vi "Actor Core.vi"(8 "error in":errorcluster, 11 "Sweeper  in":refnum<class "Sweeper.lvclass">) -> (0 "error out":errorcluster, 3 "Actor out":refnum<class "Actor.lvclass">)   [LabVIEW 2018, in "Sweeper.lvclass"]
doc: "(<B>Filename</B>: Actor Framework.lvlib:Actor.lvclass:Actor Core.vi)\n\nReceives messages to the actor, reacts to them, and initiates any error handling that may shut the actor down.\n\nDescendant classes may override this VI to append parallel tasks for the actor to complete while it handles messages. Overrides use the Call Parent Method node."
uses:
  Sweeper.lvclass
  C:/github/LabActor/Template Module/Template Module.lvclass
  C:/Program Files/National Instruments/LabVIEW 2018/vi.lib/ActorFramework/Actor/Actor.lvclass
  <vilib>/ActorFramework/Actor/Actor.lvclass
  NHMFL_Core/Libraries/Instruments/Controls/Set Output.ctl
  NHMFL_Core/Libraries/Instruments/Controls/Sweep Action.ctl
  Template Module/Template Module.lvclass/Template Module.ctl
  <vilib>/ActorFramework/Actor/Actor.lvclass/Actor.ctl
  <vilib>/ActorFramework/Message Enqueuer/Message Enqueuer.lvclass/Message Enqueuer.ctl
  NHMFL_Core/Libraries/Instruments/Results/Set Sweep/Set Sweep.lvclass
  C:/github/NHMFL_Core/Libraries/Utilities/Output Value/Output Value.lvclass
  Instrument Actor Messages/Set Output Msg/Set Output Msg.lvclass/Set Output Msg.ctl
  Template Module/Read stop event.vi
  <vilib>/ActorFramework/Message Enqueuer/Init from Existing Queue.vi
  <vilib>/ActorFramework/Message Enqueuer/Enqueue.vi
  Instrument Actor Messages/Set Output Msg/Set Output Msg.lvclass
  C:/Program Files/National Instruments/LabVIEW 2018/vi.lib/ActorFramework/Message/Message.lvclass
  <vilib>/ActorFramework/Message Priority Queue/Priority Enqueue.vi
  Instrument Actor/Instrument Actor.lvclass
  <vilib>/ActorFramework/Message Enqueuer/Message Enqueuer.lvclass
panel:
  in  "Go Button":bool
  out "Name":string
  in  "Configuration":T1={"Set point"=0.0, "Sweep rate"=0.0, "Sweep action"=enum."To set point"}
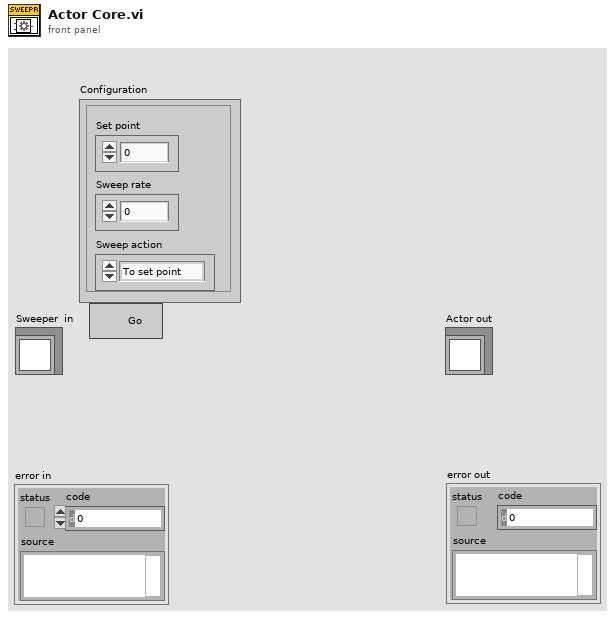
[diagram p1: front panel]
types:
  T1 = typedef "Set Output.ctl" = cluster{"Set point":dbl, "Sweep rate":dbl, "Sweep action":T2}
  T2 = typedef "Sweep Action.ctl" = enum16{"Hold", "To set point", "To zero", "Clamp"}
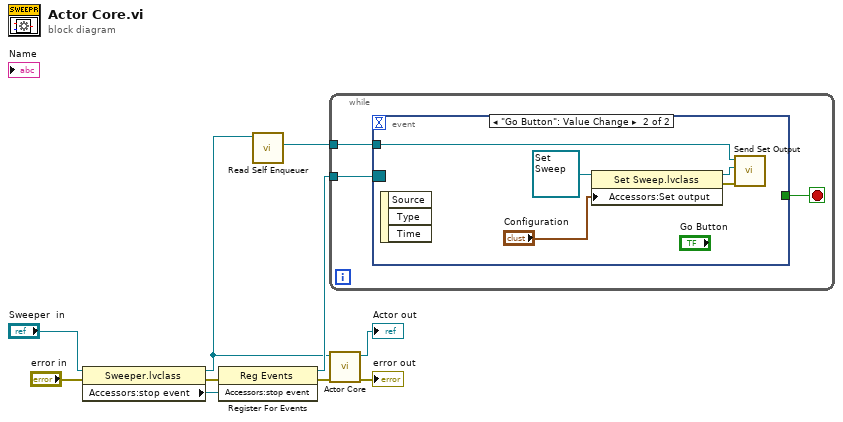
[diagram p0: block diagram]
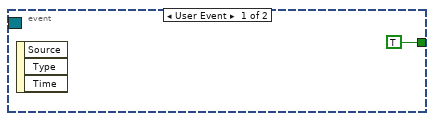
[diagram p2: hidden frame]
diagram:
  n1 = property class="Sweeper.lvclass"(reference="Sweeper  in", error in="error in") -> (reference out=w1:refnum<class "Sweeper.lvclass">, error out=w7:errorcluster, "Accessors:stop event"=w5:refnum<user-event>)
  n2 = register-events(error in=w7, w5) -> (reference out=w6:refnum<event-registration>, error out=w2:errorcluster)  [unwired: 1 in]
  n3 = call <vilib>:"Read Self Enqueuer.vi"("Actor"=w1) -> ("Self Enqueuer"=w8:refnum<class "Message Enqueuer.lvclass">)  [unwired: 10 in]
  n4 = while {
    tunnel: w6 -> [w13]
    tunnel: w8 -> [w11]
    stop <- w12 stop-if-true
    n5 = event shown="[1] \"Go Button\": Value Change" {
      selector: w13 -> [_ _]
      dyn-events: _ -> [_ _]
      timeout: _ -> [_ _]
      tunnel: [TRUE _] -> w12
      tunnel: w11 -> [_ w15]
      event User Event {
        n6 = event-data() -> ()  [unwired: 1 in, 3 out]
      }
      event "Go Button": Value Change {
        n7 = event-data() -> ()  [unwired: 1 in, 3 out]
        n8 = property class="Set Sweep.lvclass"(reference=refnum<class "Set Sweep.lvclass"> refnum ("Set Sweep.lvclass"), "Accessors:Set output"="Configuration") -> (reference out=w18:refnum<class "Set Sweep.lvclass">, error out=w17:errorcluster)  [unwired: 1 in]
        n9 = call "Send Set Output.vi"("error in (no error)"=w17, "Output value"=w18, "Message Enqueuer"=w15) -> ()  [unwired: 7 in, 2 out]
      }
    }
  }
  n10 = call-parent "Actor Core.vi"("error in"=w2, "Measure Object in"=w1) -> ("error out"=→"error out":errorcluster, "Actor out"=→"Actor out":refnum<class "Actor.lvclass">)  [unwired: 8 in]
